vi "Module Loop.vi"(8 "error in (no error)":errorcluster, 11 "Hardware Info Module in":refnum<class "Hardware Info Module.lvclass">) -> (0 "error out":errorcluster, 3 "Hardware Info Module out":refnum<class "Hardware Info Module.lvclass">)   [LabVIEW 2023, in "Volatus.lvlib" / "Hardware Info Module.lvclass"]
uses:
  Hardware Info Module.lvclass
  Module/Module.lvclass/Module.ctl
  Module/Module.lvclass
  lv-cdm/CDM-Config/Config-JSON/Config-JSON.lvclass
  Hardware Info Module.lvclass/Hardware Info Module.ctl
  StringValue/StringValue.lvclass/StringValue.ctl
  Module/Self Q.vi
  MessageQ/Delayed Send.vi
  <vilib>/Utility/error.llb/Error Cluster From Error Code.vi
  lv-promises/Promises/Promise/Promise.lvclass
  StringValue/StringValue.lvclass
  MessageQ/MessageQ.lvclass
  lv-cdm/CDM-Config/Config Manager/Config Manager.lvclass
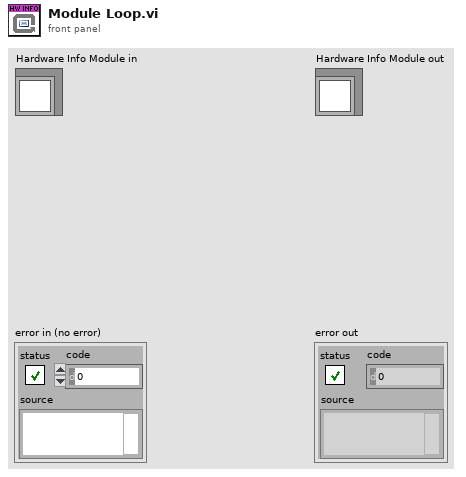
[diagram p1: front panel]
types:
  T1 = enum32{"Invalid", "Standard", "Closed", "Hidden", "Minimized", "Maximized"}
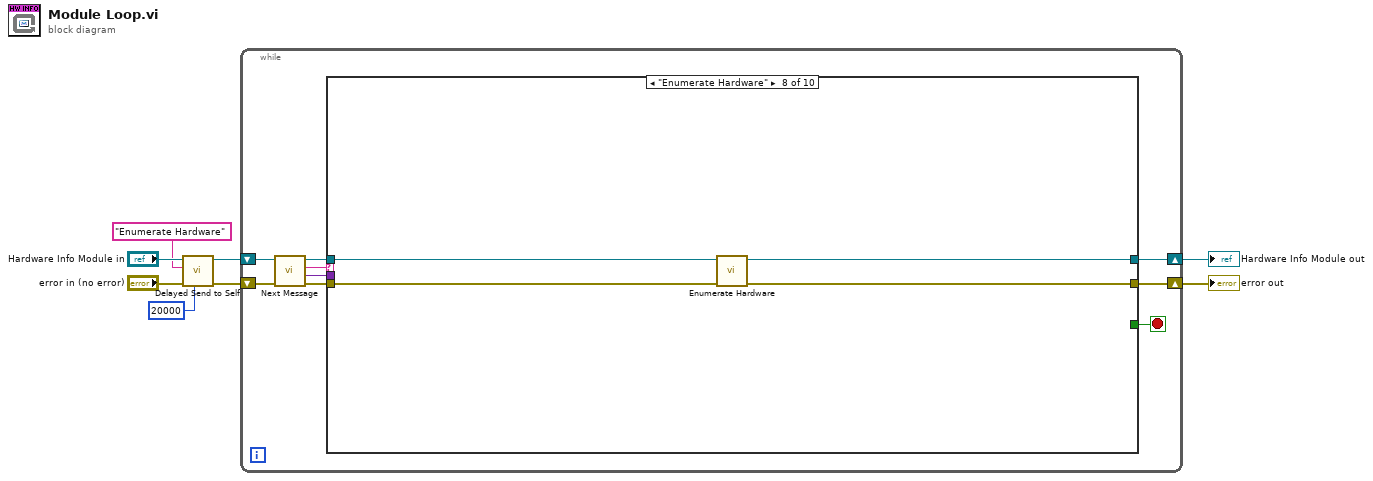
[diagram p0: block diagram]
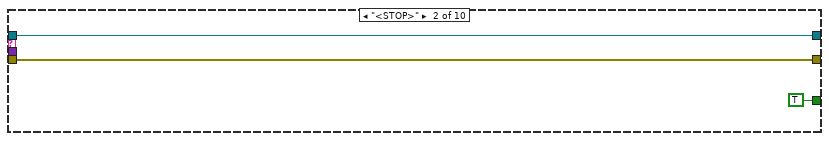
[diagram p3: hidden frame]
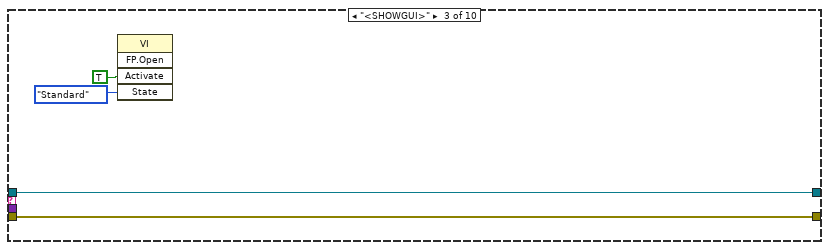
[diagram p4: hidden frame]
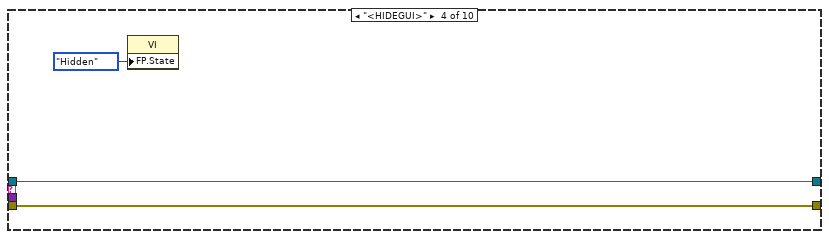
[diagram p5: hidden frame]
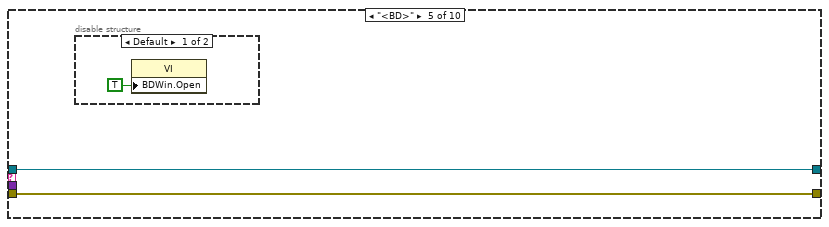
[diagram p6: hidden frame]
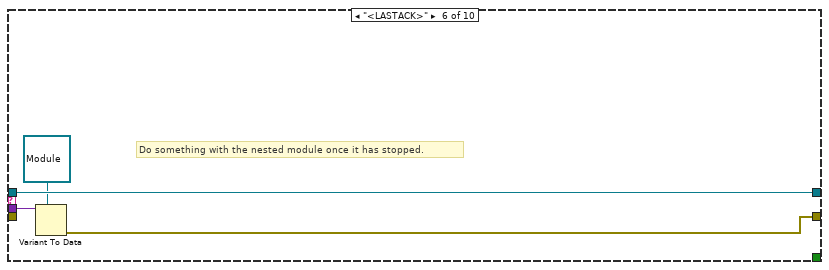
[diagram p8: hidden frame]
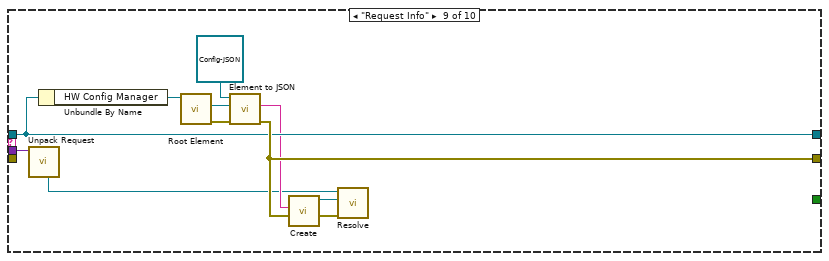
[diagram p10: hidden frame]
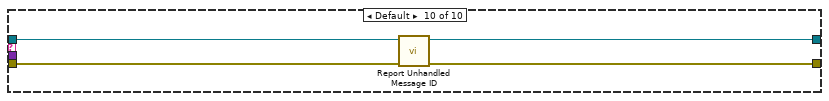
[diagram p11: hidden frame]
diagram:
  n1 = call "Delayed Send to Self.vi"("Delay ms"=20000, "error in (no error)"="error in (no error)", "Message ID"="Enumerate Hardware", "Module in"="Hardware Info Module in") -> ("error out"=w5:errorcluster, "Module out"=w3:refnum<class "Hardware Info Module.lvclass">)  [unwired: 6 in]
  n2 = while {
    shift-right: [w12] -> w6
    shift-left: w3 -> [w17]
    shift-right: [w9] -> w7
    shift-left: w5 -> [w16]
    stop <- w11 stop-if-true
    n3 = call "Next Message.vi"("error in (no error)"=w16, "Module in"=w17) -> ("error out"=w15:errorcluster, "Data"=w10:variant, "ID"=w14:string, "Module out"=w13:refnum<class "Hardware Info Module.lvclass">)  [unwired: 6 in]
    n4 = case shown="\"Enumerate Hardware\"" w14 {
      tunnel: w15 -> [w18 w20 w23 w28 w30 _ w37 w42 _ w56]
      tunnel: w13 -> [w19 w22 w26 w29 w31 w36 w38 w40 w50 w54]
      tunnel: [w19 w22 w26 w29 w31 w36 w38 w39 w50 w53] -> w12
      tunnel: [_ TRUE _ _ _ _ _ _ _ _] -> w11
      tunnel: w10 -> [_ _ _ _ _ w35 _ _ w51 _]
      tunnel: [w18 w20 w23 w28 w30 w33 w37 w41 w52 w55] -> w9
      frame "<CLOSE>" {
      }
      frame "<STOP>" {
      }
      frame "<SHOWGUI>" {
        n5 = invoke class="VI" method="FP.Open"("Activate"=TRUE ("Activate?"), "State"=T1."Standard") -> ()  [unwired: 3 in, 5 out]
      }
      frame "<HIDEGUI>" {
        n6 = property class="VI"("FP.State"=T1."Hidden" ("Front Panel Window:State")) -> ()  [unwired: 2 in, 2 out]
      }
      frame "<BD>" {
        n7 = disable-structure shown="Default" {
          frame condition #0 (active) {
            n8 = property class="VI"("BDWin.Open"=TRUE ("Block Diagram Window:Open")) -> ()  [unwired: 2 in, 2 out]
          }
          frame condition #1 {
          }
        }
      }
      frame "<LASTACK>" {
        # "Do something with the nested module once it has stopped."
        n9 = Variant To Data(type=refnum<class "Module.lvclass"> refnum ("Volatus:Module"), Variant=w35) -> (error out=w33:errorcluster)  [unwired: 1 in, 1 out]
      }
      frame "<TIMEOUT>" {
        # "No message for this module was received in time"
      }
      frame "Enumerate Hardware" {
        n10 = call "Enumerate Hardware.vi"("error in (no error)"=w42, "Hardware Info Module in"=w40) -> ("error out"=w41:errorcluster, "Hardware Info Module out"=w39:refnum<class "Hardware Info Module.lvclass">)  [unwired: 8 in]
      }
      frame "Request Info" {
        n11 = call "Unpack Request.vi"("Request Data"=w51) -> ("Promise"=w44:refnum<class "Promise.lvclass">)  [unwired: 8 in, 2 out]
        n12 = Unbundle By Name(w50) -> ("HW Config Manager"=w49:refnum<class "Config Manager.lvclass">)
        n13 = call "Root Element.vi"("Config Manager in"=w49) -> ("error out"=w47:errorcluster, "Root Element"=w48:refnum<class "Config Element.lvclass">)  [unwired: 8 in, 1 out]
        n14 = call "Element to JSON.vi"("error in (no error)"=w47, "Element"=w48, "Config-JSON"=refnum<class "Config-JSON.lvclass"> refnum) -> ("error out"=w52:errorcluster, "JSON"=w45:string)  [unwired: 7 in]
        n15 = call "Create.vi"("Value"=w45) -> ("StringValue out"=w43:refnum<class "StringValue.lvclass">)  [unwired: 10 in]
        n16 = call "Resolve.vi"("error in (no error)"=w52, "Result (None)"=w43, "Promise in"=w44) -> ()  [unwired: 7 in, 2 out]
      }
      frame Default {
        n17 = call "Report Unhandled Message ID.vi"("error in (no error)"=w56, "Module in"=w54) -> ("error out"=w55:errorcluster, "Module out"=w53:refnum<class "Hardware Info Module.lvclass">)  [unwired: 8 in]
      }
    }
  }
  "error out" <- w7
  "Hardware Info Module out" <- w6
